vi "Video Replace Dialog HTML.vi"(11 "String":string) -> (3 "appended path":path)   [LabVIEW 2017]
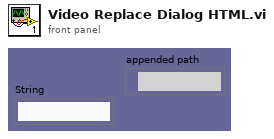
[diagram p1: front panel]
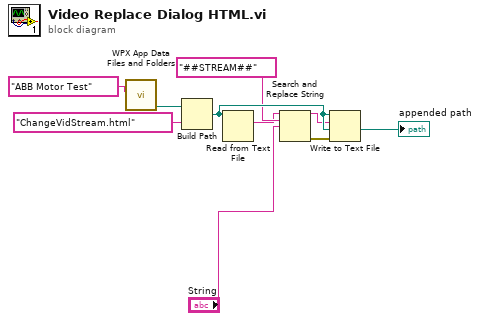
[diagram p0: block diagram]
diagram:
  n1 = call "WPX App Data Files and Folders.vi"("ApplicationName"="ABB Motor Test") -> ("DataFolder"=w1:path)  [unwired: 7 in, 3 out]
  n2 = Build Path(base path=w1, name or relative path="ChangeVidStream.html") -> (appended path=w9:path)
  "appended path" <- w9
  n3 = Read from Text File(file (use dialog)=w9) -> (text=w4:string)  [unwired: 3 in, 3 out]
  n4 = Search and Replace String(input string=w4, search string="##STREAM##", replace string="String") -> (result string=w8:string, error out=w7:errorcluster)  [unwired: 5 in, 2 out]
  n5 = Write to Text File(file (use dialog)=w9, text=w8, error in=w7) -> ()  [unwired: 1 in, 3 out]
